vi "Calc_K-P.vi"() -> ()   [LabVIEW 2020]
uses:
  <vilib>/Analysis/Matrix/Datatypes/RealMatrix.ctl
  <vilib>/Analysis/Matrix/NI_Matrix.lvlib
panel:
  in  "Number of iterations":i32=50
  in  "H Matrix":T1=[[0.0, 1.0], [9.81, 0.0]]
  in  "R Matrix":T1=[[1e-10, 0.0], [0.0, 1e-11]]
  out "Steady State Kalman Predictor Gain matrixx":T1=[[0.0001484820942425092, 0.002054458487530419], [0.9901927327955272, 0.004852302736465919]]
  out "Steady State P matrix":T1=[[2.1207340437053393e-15, 5.148482094242508e-13], [5.148482094242506e-13, 1.0099019273279553e-08]]
  in  "F  Matrix":T1=[[1.0, 0.0001], [0.0, 1.0]]
  out "Trace of P":dbl[](array[numeric])=[1.0100103864374432e-08, 1.0099071241173679e-08, 1.0099053913968777e-08, 1.0099045278716121e-08, 1.0099040091621489e-08, 1.0099036631131875e-08, 1.0099034158204801e-08, 1.0099032302912134e-08, 1.0099030859577277e-08, 1.0099029704721776e-08, 1.0099028759732476e-08, 1.0099027972181343e-08, 1.0099027305761128e-08, 1.0099026734531537e-08, 1.0099026239465627e-08, 1.0099025806290573e-08, 1.0099025424090118e-08, 1.0099025084372642e-08, 1.0099024780433431e-08, 1.0099024506908094e-08, 1.0099024259453614e-08, 1.0099024034516291e-08, 1.009902382916023e-08, 1.0099023640938665e-08, 1.009902346779618e-08, 1.009902330799346e-08, 1.009902316004879e-08, 1.0099023022692066e-08, 1.0099022894828302e-08, 1.0099022775508486e-08, 1.0099022663906008e-08, 1.0099022559297561e-08, 1.0099022461047493e-08, 1.0099022368594909e-08, 1.0099022281443006e-08, 1.0099022199150157e-08, 1.0099022121322478e-08, 1.0099022047607532e-08, 1.009902197768902e-08, 1.0099021911282272e-08, 1.0099021848130378e-08, 1.0099021788000882e-08, 1.0099021730682973e-08, 1.0099021675984975e-08, 1.0099021623732265e-08, 1.0099021573765388e-08, 1.0099021525938462e-08, 1.0099021480117755e-08, 1.0099021436180465e-08, 1.0099021394013596e-08]
  in  "Q'=GQG' (Q scalar =1)":T1=[[2.5000000000000003e-17, 5e-13], [5e-13, 1e-08]]
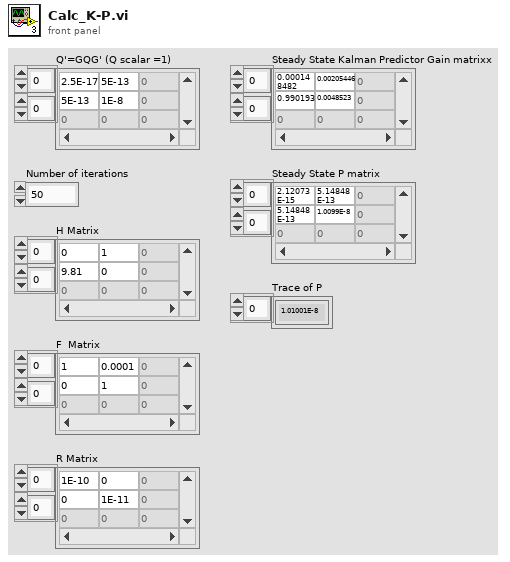
[diagram p1: front panel]
types:
  T1 = typedef "NI_Matrix.lvlib/RealMatrix.ctl" = dbl[][]
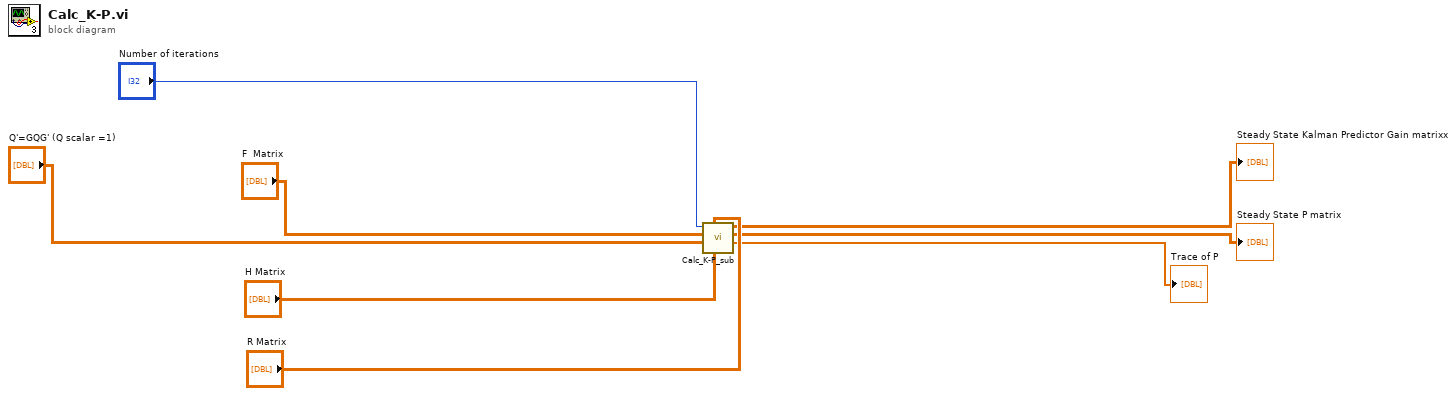
[diagram p0: block diagram]
diagram:
  n1 = call "Calc_K-P_sub.vi"("H Matrix"="H Matrix", "R Matrix"="R Matrix", "Q'=GQG' (Q scalar =1)"="Q'=GQG' (Q scalar =1)", "F  Matrix"="F  Matrix", "Number of iterations"="Number of iterations") -> ("Trace of P"=→"Trace of P":dbl[], "Steady State P matrix"=→"Steady State P matrix":T1, "Steady State Kalman Predictor Gain matrixx"=→"Steady State Kalman Predictor Gain matrixx":T1)  [unwired: 4 in]
